vi "PbDelay_1ms.vi"   [LabVIEW 2021]
doc: "1 millisecond delay\nfor settling of data"
panel:
  # "PbDelay_1ms.vi"
  # "This delay is used for ensuring that Picobus signals have reliably reached their states before reading the data or changing the state of the signal again (data integrity).  Although 1ms is the shortest delay that Windows offers, it is about ten times longer than really needed for Picobus."
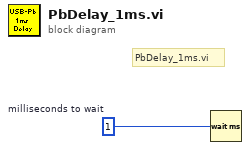
[diagram p0: block diagram]
diagram:
  w1 = u32 1  # milliseconds to wait
  # "PbDelay_1ms.vi"
  n1 = Wait (ms)(milliseconds to wait=w1) -> ()  [unwired: 1 out]
